vi "Draw Tree.vi"(8 "error in (no error)":errorcluster, 11 "Loop Data":T1) -> (0 "error out":errorcluster)   [LabVIEW 2016, in "System Mapping Tool.lvlib"]
uses:
  System Mapping Tool.lvlib
  TypeDefs/Loop Data.ctl
  TypeDefs/UI Refs.ctl
  NationalInstruments.VeriStand.SystemDefinitionAPI
  NationalInstruments.VeriStand.SystemStorageUI
  NationalInstruments.VeriStand.SystemStorage
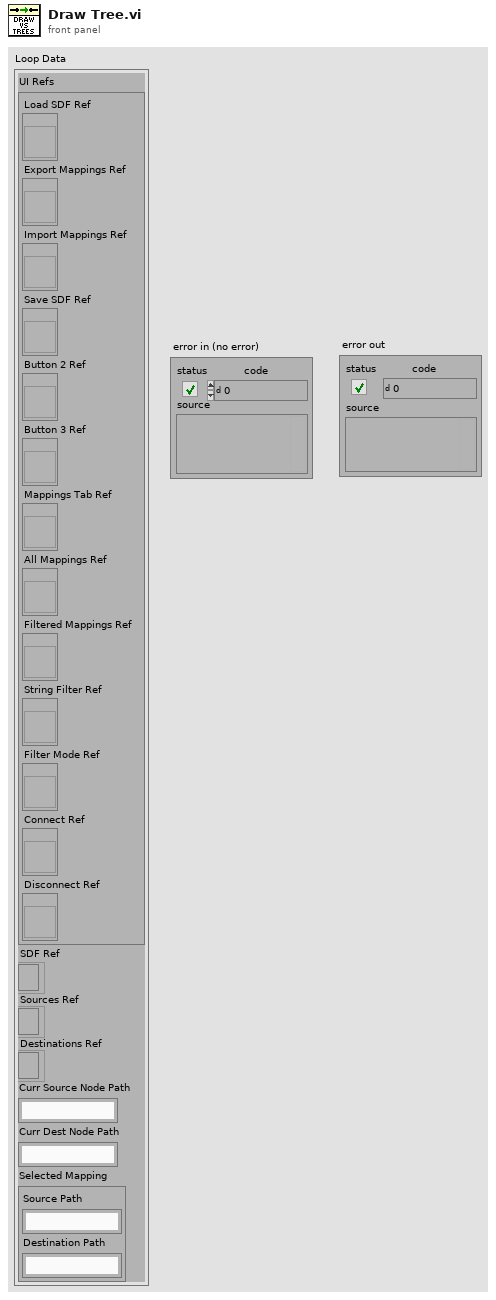
[diagram p1: front panel]
types:
  T1 = typedef "System Mapping Tool.lvlib/Loop Data.ctl" = cluster{"UI Refs":T2, "SDF Ref":refnum<k24>, "Sources Ref":refnum<k24>, "Destinations Ref":refnum<k24>, "Curr Source Node Path":string, "Curr Dest Node Path":string, "Selected Mapping":cluster{"Source Path":string, "Destination Path":string}}
  T2 = typedef "System Mapping Tool.lvlib/UI Refs.ctl" = cluster{"Load SDF Ref":refnum<vi>, "Export Mappings Ref":refnum<vi>, "Import Mappings Ref":refnum<vi>, "Save SDF Ref":refnum<vi>, "Button 2 Ref":refnum<vi>, "Button 3 Ref":refnum<vi>, "Mappings Tab Ref":refnum<vi>, "All Mappings Ref":refnum<vi>, "Filtered Mappings Ref":refnum<vi>, "String Filter Ref":refnum<vi>, "Filter Mode Ref":refnum<vi>, "Connect Ref":refnum<vi>, "Disconnect Ref":refnum<vi>}
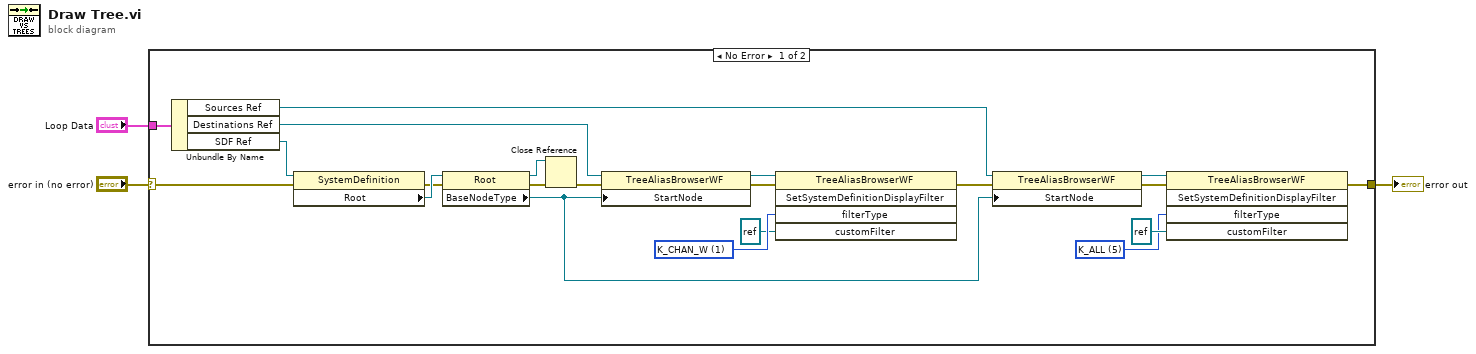
[diagram p0: block diagram]
diagram:
  n1 = case shown="No Error" "error in (no error)" {
    selector: "error in (no error)" -> [w22 w25]
    tunnel: [w4 w25] -> w2
    tunnel: "Loop Data" -> [w24 _]
    frame No Error {
      w10 = u8 5 items=["K_CHAN_R", "K_CHAN_W", "K_CHAN_RW", "K_CHAN_VOLT", "K_CHAN_FAULT", "K_ALL", "K_CUSTOM", "K_CHAN_R_VIS", "K_CHAN_W_VIS", "K_CHAN_RW_VIS", "K_CHAN_VOLT_VIS", "K_CHAN_FAULT_VIS", "K_WAVE", "K_WAVE_VIS", "K_WAVE_DBL", "K_WAVE_CDB", "K_WAVE_DBL_VIS", "K_WAVE_CDB_VIS"] ("filterType")
      w13 = u8 1 items=["K_CHAN_R", "K_CHAN_W", "K_CHAN_RW", "K_CHAN_VOLT", "K_CHAN_FAULT", "K_ALL", "K_CUSTOM", "K_CHAN_R_VIS", "K_CHAN_W_VIS", "K_CHAN_RW_VIS", "K_CHAN_VOLT_VIS", "K_CHAN_FAULT_VIS", "K_WAVE", "K_WAVE_VIS", "K_WAVE_DBL", "K_WAVE_CDB", "K_WAVE_DBL_VIS", "K_WAVE_CDB_VIS"] ("filterType")
      n2 = Unbundle By Name(w24) -> ("Sources Ref"=w6:refnum<k24>, "Destinations Ref"=w16:refnum<k24>, "SDF Ref"=w23:refnum<k24>)
      n3 = property class="SystemDefinition"(reference=w23, error in=w22) -> (error out=w20:errorcluster, "Root"=w21:refnum<k24>)  [unwired: 1 out]
      n4 = property class="Root"(reference=w21, error in=w20) -> (reference out=w18:refnum<k24>, error out=w19:errorcluster, "BaseNodeType"=w5:refnum<k24>)
      n5 = Close Reference(reference=w18, error in (no error)=w19) -> (error out=w17:errorcluster)
      n6 = property class="TreeAliasBrowserWF"(reference=w16, error in=w17, "StartNode"=w5) -> (reference out=w14:refnum<k24>, error out=w15:errorcluster)
      n7 = invoke class="TreeAliasBrowserWF" method="SetSystemDefinitionDisplayFilter"(reference=w14, error in=w15, "filterType"=w13, "customFilter"=refnum<k24> refnum) -> (error out=w7:errorcluster)  [unwired: 1 in, 4 out]
      n8 = property class="TreeAliasBrowserWF"(reference=w6, error in=w7, "StartNode"=w5) -> (reference out=w9:refnum<k24>, error out=w8:errorcluster)
      n9 = invoke class="TreeAliasBrowserWF" method="SetSystemDefinitionDisplayFilter"(reference=w9, error in=w8, "filterType"=w10, "customFilter"=refnum<k24> refnum) -> (error out=w4:errorcluster)  [unwired: 1 in, 4 out]
    }
    frame Error {
    }
  }
  "error out" <- w2
